vi "Configure Trigger Delay.vi"(8 "error in (no error)":errorcluster, 10 "Delay Time (0 s)":dbl, 11 "VISA resource name":refnum<visa-resource-name>) -> (0 "error out":errorcluster, 3 "VISA resource name out":refnum<visa-resource-name>)   [LabVIEW 2018, in "Agilent U2000 Series.lvlib"]
doc: "Set the delay between the delayed trigger point and the start of the trace for the U2040 X-Series.\n\nNote: \n(1) This VI is only applicable for U2042XA/U2044XA/U2049XA.\n(2) Measurement function configured in <b>Configure Measurement.vi</b> should be set to Normal. If the measurement function is set to Average, an error -221, \"Settings conflict\" will occur."
uses:
  Agilent U2000 Series.lvlib
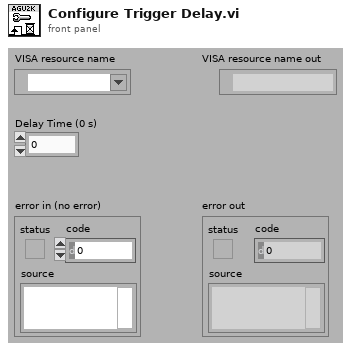
[diagram p1: front panel]
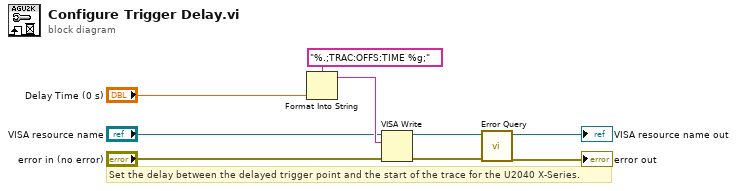
[diagram p0: block diagram]
diagram:
  # "Set the delay between the delayed trigger point and the start of the trace for the U2040 X-Series."
  n1 = Format Into String(format string="%.;TRAC:OFFS:TIME %g;", "Delay Time (0 s)") -> (resulting string=w7:string)  [unwired: 2 in, 1 out]
  n2 = VISA Write(VISA resource name="VISA resource name", write buffer=w7, error in (no error)="error in (no error)") -> (VISA resource name out=w4:refnum<visa-resource-name>, error out=w3:errorcluster)  [unwired: 1 out]
  n3 = call "Error Query.vi"("error in (no error)"=w3, "VISA resource name"=w4) -> ("error out"=→"error out":errorcluster, "VISA resource name out"=→"VISA resource name out":refnum<visa-resource-name>)  [unwired: 6 in, 2 out]
